vi "Read Action VI Properties.vi"(8 "error in (no error)":errorcluster, 11 "ActionVI in":refnum<class "ActionVI.lvclass">) -> (0 "error out":errorcluster, 2 "Path":T1, 3 "ActionVI out":refnum<class "ActionVI.lvclass">)   [LabVIEW 2019, in "ActionVI.lvclass"]
uses:
  ActionVI.lvclass
  XML Controls/Path Cluster.ctl
  ActionVI.lvclass/ActionVI.ctl
  VeriStand Custom Device XML Parser.lvlib
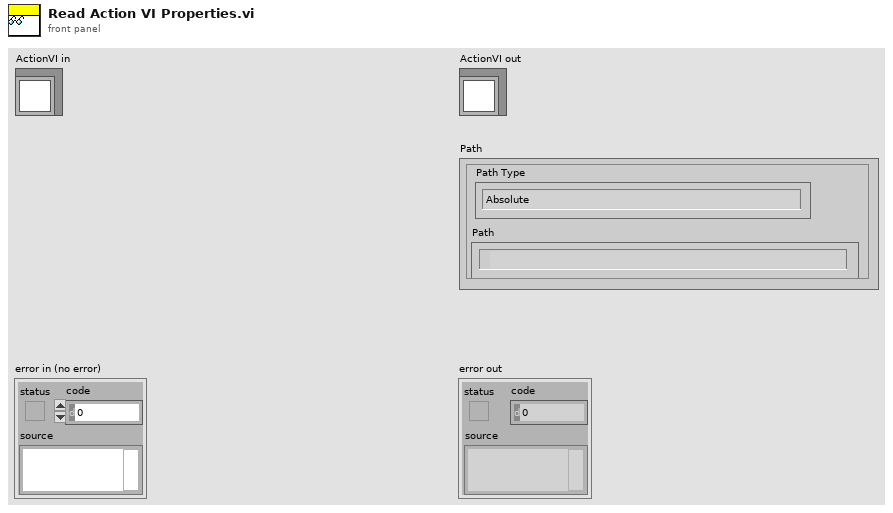
[diagram p1: front panel]
types:
  T1 = typedef "VeriStand Custom Device XML Parser.lvlib/Path Cluster.ctl" = cluster{"Path":path, "Path Type":enum16{"Absolute", "To Base", "To Common Doc Dir", "To Application Data Dir"}}
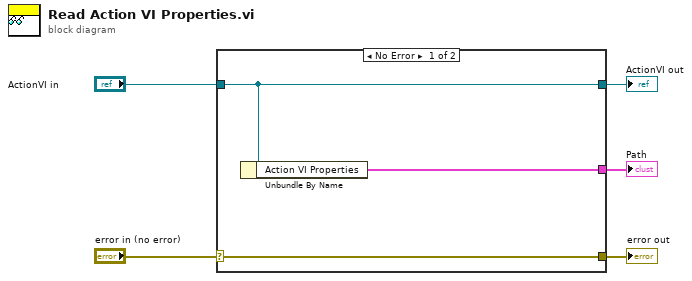
[diagram p0: block diagram]
diagram:
  n1 = case shown="No Error" "error in (no error)" {
    selector: "error in (no error)" -> [w8 w9]
    tunnel: [w8 w9] -> w4
    tunnel: [w7 w10] -> w2
    tunnel: "ActionVI in" -> [w7 w10]
    tunnel: [w6 _] -> w1
    frame No Error {
      n2 = Unbundle By Name(w7) -> ("Action VI Properties"=w6:T1)
    }
    frame Error {
    }
  }
  "error out" <- w4
  "ActionVI out" <- w2
  "Path" <- w1
